vi "Parallelschaltung.vi"(2 "error in (no error)":errorcluster, 3 "Array In":dbl[](array[numeric])) -> (0 "error out":errorcluster, 1 "Out":dbl)   [LabVIEW 2022 SP3]
uses:
  <vilib>/Utility/error.llb/Error Cluster From Error Code.vi
  <vilib>/ErrorRing/Error Ring.xnode
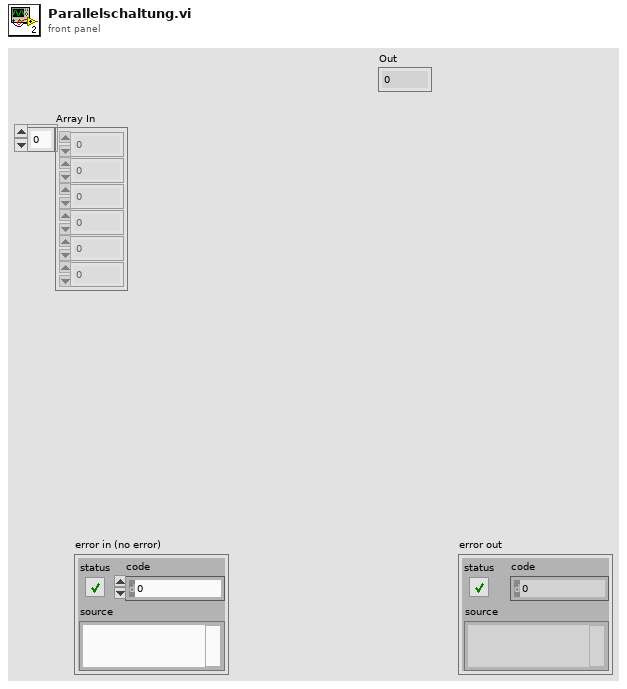
[diagram p1: front panel]
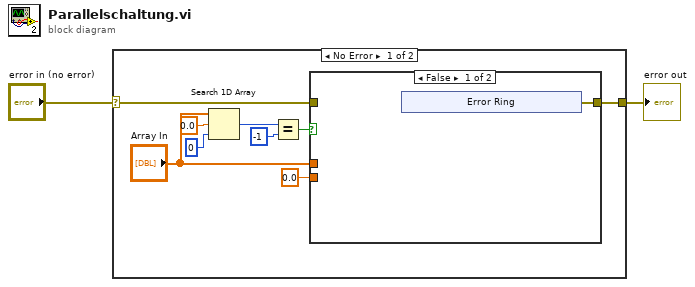
[diagram p0: block diagram]
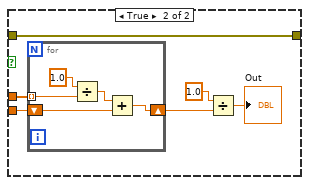
[diagram p2: hidden frame]
diagram:
  n1 = case shown="No Error" "error in (no error)" {
    selector: "error in (no error)" -> [w3 w29]
    tunnel: [w5 w29] -> w1
    frame No Error {
      n2 = Search 1D Array(1D array="Array In", element=0.0, start index (0)=0) -> (index of element=w8:i32)
      n3 = Equal?(x=w8, y=-1) -> (x = y?=w6:bool)
      n4 = case shown="False" w6 {
        tunnel: 0.0 -> [_ w23]
        tunnel: [w12 w21] -> w5
        tunnel: "Array In" -> [_ w22]
        tunnel: w3 -> [_ w21]
        frame False {
          n5 = xnode "Error Ring"() -> ("error out"=w12:errorcluster)
        }
        frame True {
          n6 = for {
            shift-right: [w25] -> w19
            shift-left: w23 -> [w26]
            tunnel: w22 -> [w24] mode=indexing
            n7 = Divide(x=1.0, y=w24) -> (x/y=w27:dbl)
            n8 = Add(x=w27, y=w26) -> (x+y=w25:dbl)
          }
          n9 = Divide(x=1.0, y=w19) -> (x/y=→"Out":dbl)
        }
      }
    }
    frame Error {
    }
  }
  "error out" <- w1
